vi "Unregister.vi"(0 "BroadcastRegistry In":T1, 5 "Status":string, 7 "Source":string, 9 "Api":string="api", 11 "Target":string) -> (4 "BroadcastRegistry Out":T1)   [LabVIEW 2017, in "Communicable State Machine.lvlib"]
doc: "### Unregister.vi\n\n-- <b>Controls</b> --\n- <b>BroadcastRegistry in</b>:\n- <b>Status</b>:\n- <b>Source</b>:\n- <b>api</b>:\n- <b>Target</b>:\n\n-- <b>Indicators</b> --\n- <b>BroadcastRegistry out</b>:"
uses:
  Communicable State Machine.lvlib
  BroadcastRegistry.ctl
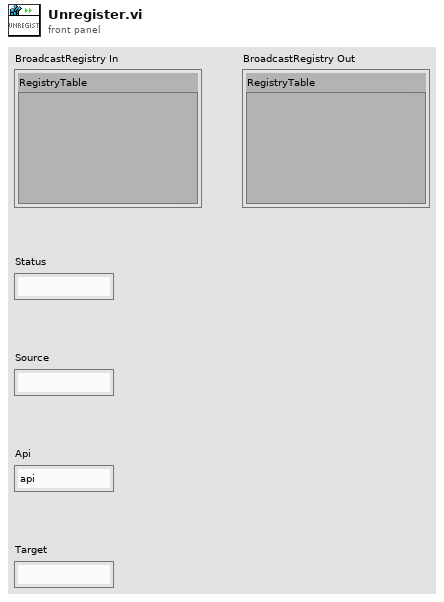
[diagram p1: front panel]
types:
  T1 = typedef "Communicable State Machine.lvlib/BroadcastRegistry.ctl" = cluster{"RegistryTable":variant}
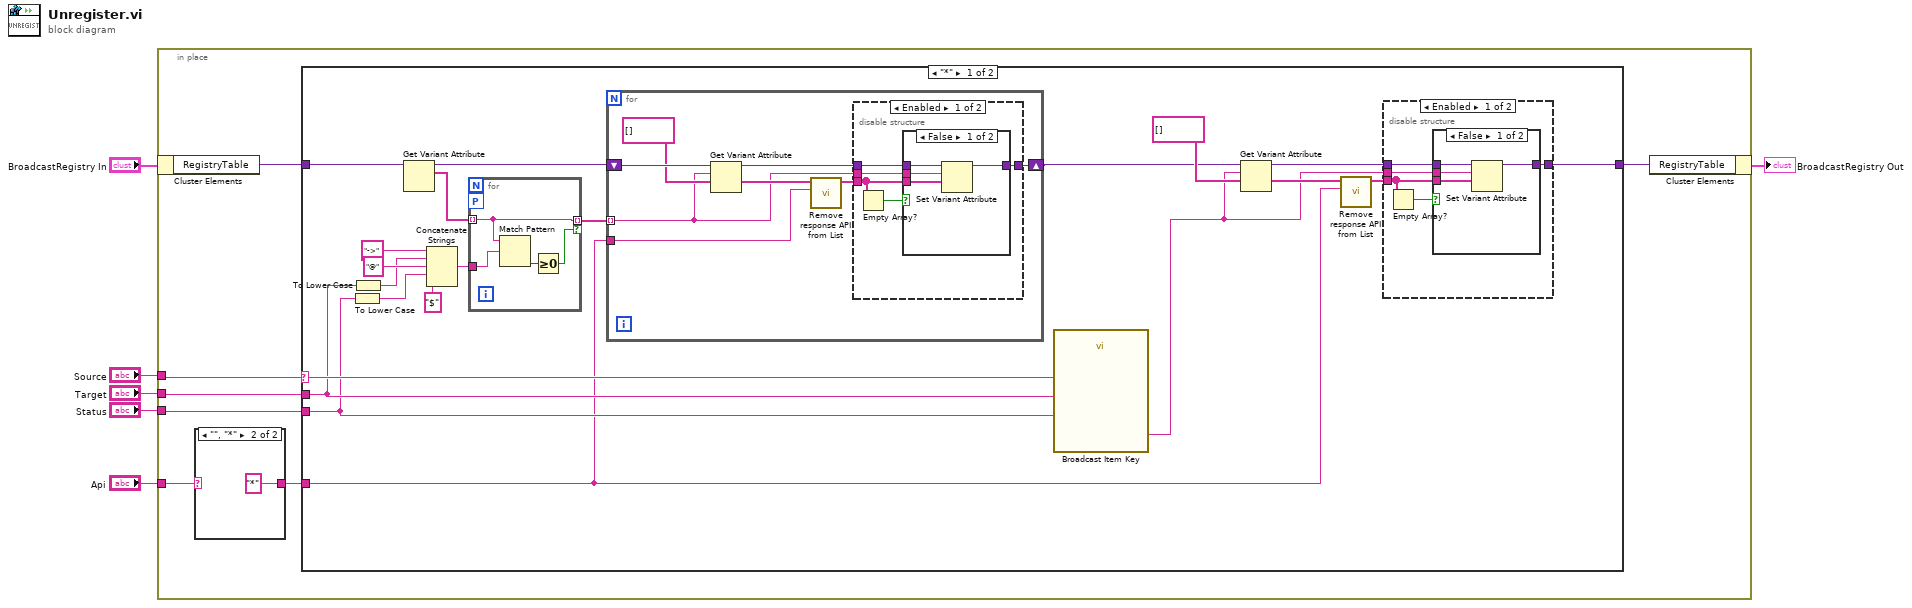
[diagram p0: block diagram]
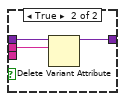
[diagram p2: hidden frame]
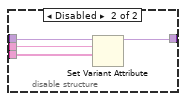
[diagram p3: hidden frame]
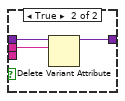
[diagram p4: hidden frame]
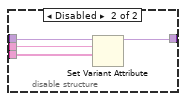
[diagram p5: hidden frame]
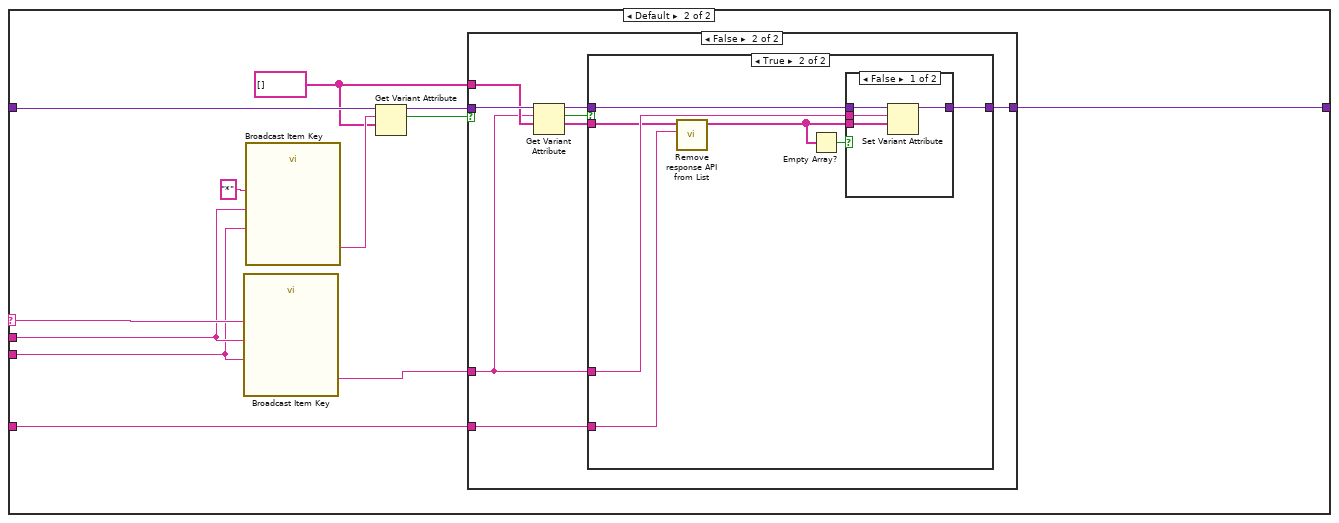
[diagram p6: hidden frame]
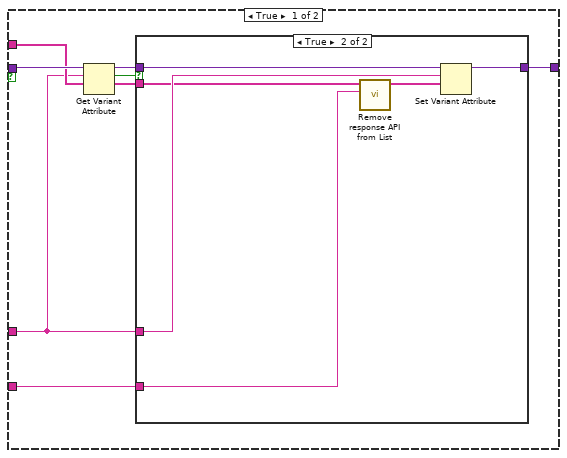
[diagram p7: hidden frame]
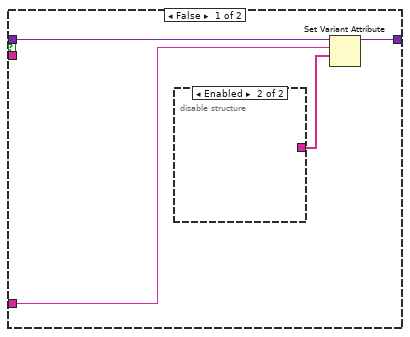
[diagram p8: hidden frame]
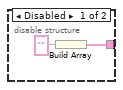
[diagram p9: hidden frame]
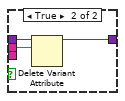
[diagram p11: hidden frame]
diagram:
  n1 = in-place {
    in-place-border: "Status" -> [w9]
    in-place-border: "Target" -> [w10]
    in-place-border: "Source" -> [w11]
    in-place-border: "Api" -> [w8]
    n2 = in-place-cluster #1("BroadcastRegistry In") -> ("RegistryTable"=w13:variant)
    n3 = case shown="\"\", \"*\"" w8 {
      selector: w8 -> [w134 _]
      tunnel: [w134 "*"] -> w7
      frame Default {
      }
      frame "", "*" {
      }
    }
    n4 = case shown="\"*\"" w11 {
      selector: w11 -> [w34 w84]
      tunnel: w13 -> [w26 w88]
      tunnel: [w17 w90] -> w12
      tunnel: w10 -> [w25 w83]
      tunnel: w9 -> [w24 w82]
      tunnel: w7 -> [w14 w79]
      frame "*" {
        n5 = To Lower Case(string=w24) -> (all lower case string=w27:string)
        n6 = To Lower Case(string=w25) -> (all lower case string=w29:string)
        n7 = Get Variant Attribute(Variant=w26) -> (duplicate Variant=w33:variant, names=w32:string[])  [unwired: 3 in, 2 out]
        n8 = Concatenate Strings("->" ("string"), w29, "@" ("string"), w27, "$" ("string")) -> (w22:string)
        n9 = for {
          tunnel: w32 -> [w78] mode=indexing
          tunnel: [w78] -> w28 mode=indexing if=w75
          tunnel: w22 -> [w77]
          workers-P: _ -> [_]
          n10 = Match Pattern(string=w78, regular expression=w77) -> (offset past match=w76:i32)  [unwired: 1 in, 3 out]
          n11 = Greater Or Equal To 0?(x=w76) -> (x >= 0?=w75:bool)
        }
        n12 = for {
          shift-right: [w53] -> w16
          shift-left: w33 -> [w58]
          tunnel: w28 -> [w51] mode=indexing
          tunnel: w14 -> [w56]
          n13 = Get Variant Attribute(Variant=w58, name=w51, default value (empty Variant)=string[] [] ("string")) -> (duplicate Variant=w54:variant, value=w55:string[])  [unwired: 1 in, 2 out]
          n14 = call "Remove response API from List.vi"("API"=w56, "Output Cluster In"=w55) -> ("Output Cluster Out"=w52:string[])  [unwired: 9 in]
          n15 = disable-structure shown="Enabled" {
            disable-tunnel: w54 -> [w62 w73]
            disable-tunnel: [w61 w71] -> w53
            disable-tunnel: w52 -> [w60 w72]
            disable-tunnel: w51 -> [w59 w74]
            frame Enabled {
              n16 = Empty Array?(array=w60) -> (empty?=w63:bool)
              n17 = case shown="False" w63 {
                tunnel: [w67 w70] -> w61
                tunnel: w62 -> [w66 w69]
                tunnel: w60 -> [w65 _]
                tunnel: w59 -> [w64 w68]
                frame False {
                  n18 = Set Variant Attribute(Variant=w66, name=w64, value=w65) -> (Variant out=w67:variant)  [unwired: 1 in, 2 out]
                }
                frame True {
                  n19 = Delete Variant Attribute(6:w68, 7:w69) -> (3:w70:variant)  [unwired: 1 in, 2 out]
                }
              }
            }
            frame Disabled {
              n20 = Set Variant Attribute(Variant=w73, name=w74, value=w72) -> (Variant out=w71:variant)  [unwired: 1 in, 2 out]
            }
          }
        }
        n21 = call "Broadcast Item Key.vi"("Status"=w24, "Target"=w25, "Source"=w34) -> ("Key"=w15:string)  [unwired: 2 in]
        n22 = Get Variant Attribute(Variant=w16, name=w15, default value (empty Variant)=string[] [] ("string")) -> (duplicate Variant=w19:variant, value=w20:string[])  [unwired: 1 in, 2 out]
        n23 = call "Remove response API from List.vi"("API"=w14, "Output Cluster In"=w20) -> ("Output Cluster Out"=w18:string[])  [unwired: 9 in]
        n24 = disable-structure shown="Enabled" {
          disable-tunnel: w19 -> [w38 w49]
          disable-tunnel: [w37 w47] -> w17
          disable-tunnel: w18 -> [w36 w48]
          disable-tunnel: w15 -> [w35 w50]
          frame Enabled {
            n25 = Empty Array?(array=w36) -> (empty?=w39:bool)
            n26 = case shown="False" w39 {
              tunnel: [w43 w46] -> w37
              tunnel: w38 -> [w42 w45]
              tunnel: w36 -> [w41 _]
              tunnel: w35 -> [w40 w44]
              frame False {
                n27 = Set Variant Attribute(Variant=w42, name=w40, value=w41) -> (Variant out=w43:variant)  [unwired: 1 in, 2 out]
              }
              frame True {
                n28 = Delete Variant Attribute(6:w44, 7:w45) -> (3:w46:variant)  [unwired: 1 in, 2 out]
              }
            }
          }
          frame Disabled {
            n29 = Set Variant Attribute(Variant=w49, name=w50, value=w48) -> (Variant out=w47:variant)  [unwired: 1 in, 2 out]
          }
        }
      }
      frame Default {
        w80 = string[] [] ("output cluster")
        n30 = call "Broadcast Item Key.vi"("Status"=w82, "Target"=w83, "Source"=w84) -> ("Key"=w81:string)  [unwired: 2 in]
        n31 = call "Broadcast Item Key.vi"("Status"=w82, "Target"=w83, "Source"="*") -> ("Key"=w86:string)  [unwired: 2 in]
        n32 = Get Variant Attribute(Variant=w88, name=w86, default value (empty Variant)=w80) -> (duplicate Variant=w87:variant, found=w85:bool)  [unwired: 1 in, 2 out]
        n33 = case shown="False" w85 {
          tunnel: [w98 w118] -> w90
          tunnel: w87 -> [w97 w117]
          tunnel: w81 -> [w94 w114]
          tunnel: w80 -> [w95 w115]
          tunnel: w79 -> [w91 w112]
          frame True {
            n34 = Get Variant Attribute(Variant=w97, name=w94, default value (empty Variant)=w95) -> (duplicate Variant=w96:variant, found=w93:bool, value=w92:string[])  [unwired: 1 in, 1 out]
            n35 = case shown="True" w93 {
              tunnel: [w102 w110] -> w98
              tunnel: w96 -> [w100 w109]
              tunnel: w94 -> [w99 w108]
              tunnel: w92 -> [_ w106]
              tunnel: w91 -> [_ w107]
              frame False {
                n36 = disable-structure shown="Enabled" {
                  disable-tunnel: [w104 _] -> w101
                  frame Disabled {
                    n37 = Build Array("" ("response message")) -> (w104:string[])
                  }
                  frame Enabled {
                  }
                }
                n38 = Set Variant Attribute(Variant=w100, name=w99, value=w101) -> (Variant out=w102:variant)  [unwired: 1 in, 2 out]
              }
              frame True {
                n39 = call "Remove response API from List.vi"("API"=w107, "Output Cluster In"=w106) -> ("Output Cluster Out"=w105:string[])  [unwired: 9 in]
                n40 = Set Variant Attribute(Variant=w109, name=w108, value=w105) -> (Variant out=w110:variant)  [unwired: 1 in, 2 out]
              }
            }
          }
          frame False {
            n41 = Get Variant Attribute(Variant=w117, name=w114, default value (empty Variant)=w115) -> (duplicate Variant=w116:variant, found=w111:bool, value=w113:string[])  [unwired: 1 in, 1 out]
            n42 = case shown="True" w111 {
              tunnel: [w119 w126] -> w118
              tunnel: w116 -> [w119 w125]
              tunnel: w114 -> [_ w124]
              tunnel: w113 -> [_ w121]
              tunnel: w112 -> [_ w120]
              frame False {
              }
              frame True {
                n43 = call "Remove response API from List.vi"("API"=w120, "Output Cluster In"=w121) -> ("Output Cluster Out"=w123:string[])  [unwired: 9 in]
                n44 = Empty Array?(array=w123) -> (empty?=w122:bool)
                n45 = case shown="False" w122 {
                  tunnel: [w130 w132] -> w126
                  tunnel: w125 -> [w129 w133]
                  tunnel: w124 -> [w128 w131]
                  tunnel: w123 -> [w127 _]
                  frame False {
                    n46 = Set Variant Attribute(Variant=w129, name=w128, value=w127) -> (Variant out=w130:variant)  [unwired: 1 in, 2 out]
                  }
                  frame True {
                    n47 = Delete Variant Attribute(6:w131, 7:w133) -> (3:w132:variant)  [unwired: 1 in, 2 out]
                  }
                }
              }
            }
          }
        }
      }
    }
    n48 = in-place-cluster #1("RegistryTable"=w12) -> (→"BroadcastRegistry Out":T1)
  }
